vi "Write Status.vi"(8 "error in (no error)":errorcluster, 10 "Status":bool, 11 "SolarShutt in":refnum<class "SolarShutt.lvclass">) -> (0 "error out":errorcluster, 3 "SolarShutt out":refnum<class "SolarShutt.lvclass">)   [LabVIEW 2016, in "SolarShutt.lvclass"]
uses:
  SolarShutt.lvclass
  Shutter.lvclass
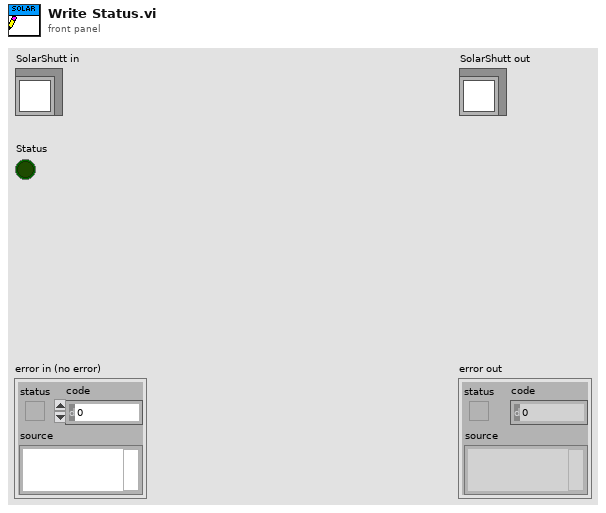
[diagram p1: front panel]
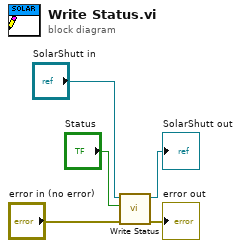
[diagram p0: block diagram]
diagram:
  n1 = call-parent "Write Status.vi"("error in (no error)"="error in (no error)", "Status"="Status", "Shutter in"="SolarShutt in") -> ("error out"=→"error out":errorcluster, "Shutter out"=→"SolarShutt out":refnum<class "SolarShutt.lvclass">)  [unwired: 7 in]
